vi "channel-Informations.vi"(0 "Channel Name":string) -> (1 "Match:":i32, 2 "No. of channels:":i32, 3 "Channel Informations:":string)   [LabVIEW 2018]
doc: "This VI uses the Physical channel as its input and determines the channels used and the total no. of channels used in data acquisition.\n\nThe output is in string format. This may be written into a file for future references.\n\n\nCreated by Vijay P. Ramalingam. July, 2006 -->virjay@olemiss.edu<--"
panel:
  # "The input which is Channel name is obtained from Physical Channel's Property node."
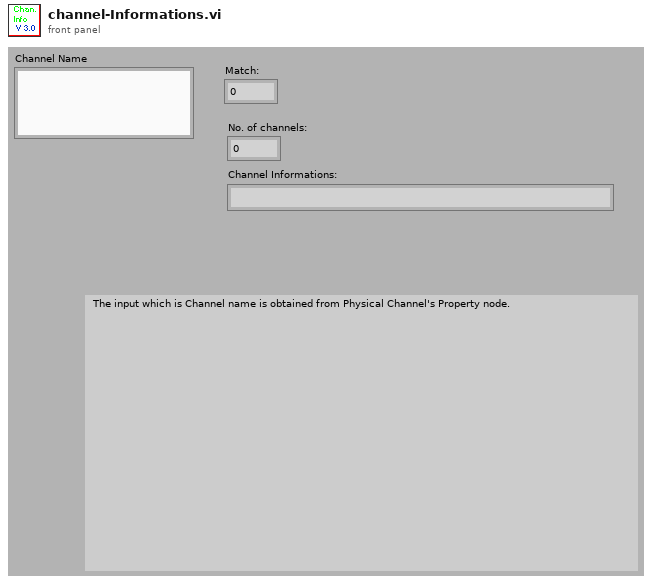
[diagram p1: front panel]
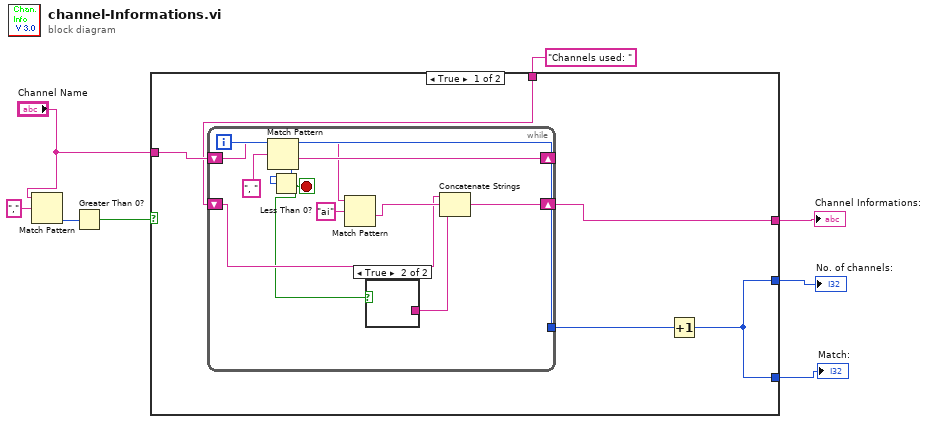
[diagram p0: block diagram]
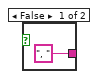
[diagram p2: hidden frame]
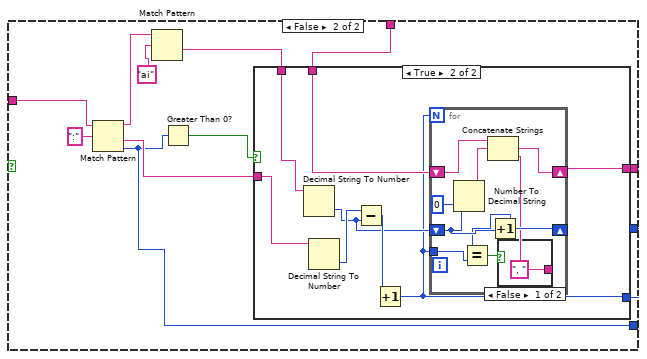
[diagram p3: hidden frame]
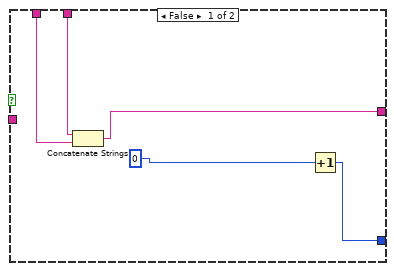
[diagram p4: hidden frame]
diagram:
  n1 = Match Pattern(string="Channel Name", regular expression=",") -> (offset past match=w7:i32)  [unwired: 1 in, 3 out]
  n2 = Greater Than 0?(x=w7) -> (x > 0?=w6:bool)
  n3 = case shown="True" w6 {
    tunnel: "Channel Name" -> [w13 w31]
    tunnel: [w9 w28] -> w5
    tunnel: [w11 w30] -> w4
    tunnel: [w9 w29] -> w3
    tunnel: "Channels used: " ("string") -> [w12 w27]
    frame True {
      n4 = while {
        tunnel: [w24] -> w10
        shift-right: [w22] -> _
        shift-left: w13 -> [w23]
        shift-right: [w17] -> w11
        shift-left: w12 -> [w16]
        i -> [w24]
        stop <- w15 stop-if-true
        n5 = Match Pattern(string=w23, regular expression=", ") -> (before substring=w21:string, after substring=w22:string, offset past match=w25:i32)  [unwired: 1 in, 1 out]
        n6 = Less Than 0?(x=w25) -> (x < 0?=w15:bool)
        n7 = Match Pattern(string=w21, regular expression="ai") -> (after substring=w19:string)  [unwired: 1 in, 3 out]
        n8 = case shown="True" w15 {
          tunnel: [", " ("regular expression") _] -> w14
          frame False {
          }
          frame True {
          }
        }
        n9 = Concatenate Strings(w16, w19, w14) -> (w17:string)
      }
      n10 = Increment(x=w10) -> (x+1=w9:i32)
    }
    frame False {
      n11 = Match Pattern(string=w31, regular expression=":") -> (before substring=w36:string, after substring=w32:string, offset past match=w29:i32)  [unwired: 1 in, 1 out]
      n12 = Match Pattern(string=w36, regular expression="ai") -> (after substring=w33:string)  [unwired: 1 in, 3 out]
      n13 = Greater Than 0?(x=w29) -> (x > 0?=w34:bool)
      n14 = case shown="True" w34 {
        tunnel: [w40 w44] -> w30
        tunnel: w33 -> [w41 w50]
        tunnel: w32 -> [_ w49]
        tunnel: [w38 w43] -> w28
        tunnel: w27 -> [w42 w45]
        frame False {
          n15 = Concatenate Strings(w42, w41) -> (w40:string)
          n16 = Increment(x=0) -> (x+1=w38:i32)
        }
        frame True {
          n17 = Decimal String To Number(string=w50) -> (number=w46:i32)  [unwired: 2 in, 1 out]
          n18 = Decimal String To Number(string=w49) -> (number=w48:i32)  [unwired: 2 in, 1 out]
          n19 = Subtract(x=w48, y=w46) -> (x-y=w47:i32)
          n20 = Increment(x=w47) -> (x+1=w43:i32)
          n21 = for {
            N: w43 -> [_]
            shift-right: [w59] -> w44
            shift-left: w45 -> [w55]
            shift-right: [w53] -> _
            shift-left: w46 -> [w58]
            tunnel: w43 -> [w54]
            n22 = Number To Decimal String(number=w58, width (-)=i16 0) -> (decimal integer string=w56:string)
            n23 = Increment(x=w58) -> (x+1=w53:i32)
            n24 = Equal?(x=w53, y=w54) -> (x = y?=w52:bool)
            n25 = case shown="False" w52 {
              tunnel: [", " ("string") _] -> w51
              frame False {
              }
              frame True {
              }
            }
            n26 = Concatenate Strings(w55, w56, w51) -> (w59:string)
          }
        }
      }
    }
  }
  "Channel Informations:" <- w4
  "No. of channels:" <- w5
  "Match:" <- w3
